vi "RSZVB Get Fixed Frequency To Signal.vi"(8 "error in (no error)":errorcluster {"code" format="%.0x"}, 9 "Signal (RF)":i32(ring) items=["RF"=0, "IF"=2, "LO 1"=3, "LO 2"=4], 10 "Channel (1)":i32=1, 11 "VISA resource name":refnum<visa-resource-name>) -> (0 "error out":errorcluster {"code" format="%.0x"}, 2 "Fixed Frequency":dbl format="%^.3e", 3 "VISA resource name out":refnum<visa-resource-name>)   [LabVIEW 2011]
doc: "This VI returns a fixed frequency at selected signal type (RF, LO 1, LO 2, or the IF signal). \n\nRemote-control command(s):\n[SENSe<Ch>:]FREQuency:CONVersion:MIXer:MFFixed? RF | LO | LO1 | LO2 | IF"
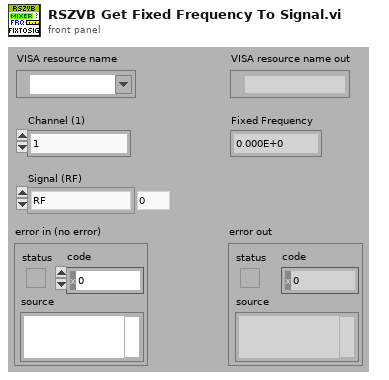
[diagram p1: front panel]
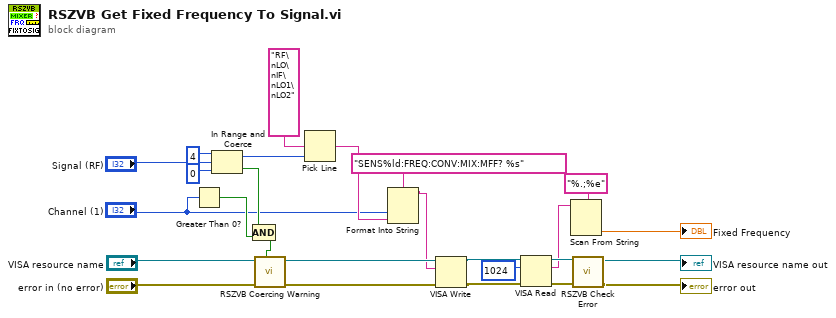
[diagram p0: block diagram]
diagram:
  n1 = Greater Than 0?(x="Channel (1)") -> (x > 0?=w17:bool)
  n2 = In Range and Coerce(upper limit=4, x="Signal (RF)", lower limit=0) -> (coerced(x)=w20:i32, In Range?=w15:bool)
  n3 = Compound Arithmetic op=AND(w15, w17) -> (w24:bool)
  n4 = call "RSZVB Coercing Warning.vi"("In Range?"=w24, "error in (no error)"="error in (no error)", "VISA session"="VISA resource name") -> ("error out"=w25:errorcluster, "dup VISA session"=w26:refnum<visa-resource-name>)  [unwired: 7 in]
  n5 = Pick Line(multi-line string="RF\nLO\nIF\nLO1\nLO2", line index=w20) -> (output string=w16:string)  [unwired: 1 in]
  n6 = Format Into String(format string="SENS%ld:FREQ:CONV:MIX:MFF? %s", "Channel (1)", w16) -> (resulting string=w22:string)  [unwired: 2 in, 1 out]
  n7 = VISA Write(VISA resource name=w26, write buffer=w22, error in (no error)=w25) -> (VISA resource name out=w13:refnum<visa-resource-name>, error out=w12:errorcluster)  [unwired: 1 out]
  n8 = VISA Read(VISA resource name=w13, byte count=u32 1024 ("byte count (0)"), error in (no error)=w12) -> (VISA resource name out=w11:refnum<visa-resource-name>, read buffer=w8:string, error out=w10:errorcluster)  [unwired: 1 out]
  n9 = Scan From String(format string="%.;%e", input string=w8) -> (output 1=→"Fixed Frequency":dbl)  [unwired: 3 in, 3 out]
  n10 = call "RSZVB Check Error.vi"("error in (no error)"=w10, "VISA session"=w11) -> ("error out"=→"error out":errorcluster, "dup VISA session"=→"VISA resource name out":refnum<visa-resource-name>)  [unwired: 8 in]
